vi "Delete Mapping.vi"(8 "error in (no error)":errorcluster, 10 "Destination Path":string, 11 "SDF Ref":refnum<k24>) -> (0 "error out":errorcluster)   [LabVIEW 2016, in "System Mapping Tool.lvlib"]
uses:
  System Mapping Tool.lvlib
  NationalInstruments.VeriStand.SystemDefinitionAPI
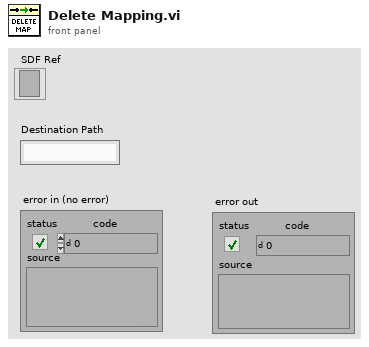
[diagram p1: front panel]
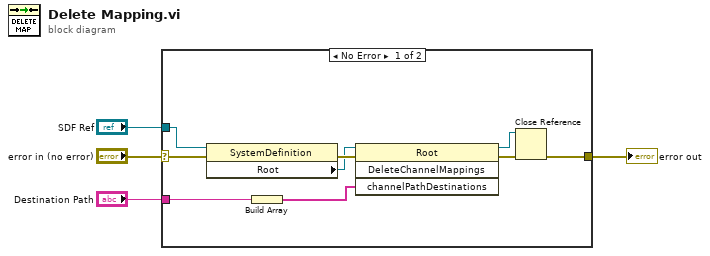
[diagram p0: block diagram]
diagram:
  n1 = case shown="No Error" "error in (no error)" {
    selector: "error in (no error)" -> [w9 w14]
    tunnel: [w8 w14] -> w3
    tunnel: "SDF Ref" -> [w7 _]
    tunnel: "Destination Path" -> [w6 _]
    frame No Error {
      n2 = property class="SystemDefinition"(reference=w7, error in=w9) -> (error out=w13:errorcluster, "Root"=w12:refnum<k24>)  [unwired: 1 out]
      n3 = Build Array(w6) -> (w5:string[])
      n4 = invoke class="Root" method="DeleteChannelMappings"(reference=w12, error in=w13, "channelPathDestinations"=w5) -> (reference out=w10:refnum<k24>, error out=w11:errorcluster)  [unwired: 1 in, 2 out]
      n5 = Close Reference(reference=w10, error in (no error)=w11) -> (error out=w8:errorcluster)
    }
    frame Error {
    }
  }
  "error out" <- w3
